vi "Load DAC Configuration.vi"(8 "error in":errorcluster, 10 "Config File refnum in":T1, 11 "DAC Keller Diff P 23X in":refnum<class "DAC Keller Diff P 23X.lvclass">) -> (0 "error out":errorcluster, 2 "Config File refnum out":T1, 3 "DAC Keller Diff P 23X out":refnum<class "DAC Keller Diff P 23X.lvclass">)   [LabVIEW 2019, in "DAC.lvlib" / "DAC Keller Diff P 23X.lvclass"]
uses:
  DAC Keller Diff P 23X.lvclass
  C:/Users/krio/Documents/LV_Projects/test-stand/App/DAC/DAC.lvclass
  <vilib>/Utility/config.llb/Config Data RefNum.ctl
  DAC.lvclass/DAC.ctl
  DAC Keller Diff P 23X.lvclass/DAC Keller Diff P 23X.ctl
  <vilib>/Utility/config.llb/Read Key (String).vi
  DAC.lvclass
  <vilib>/Utility/config.llb/NI_LVConfig.lvlib
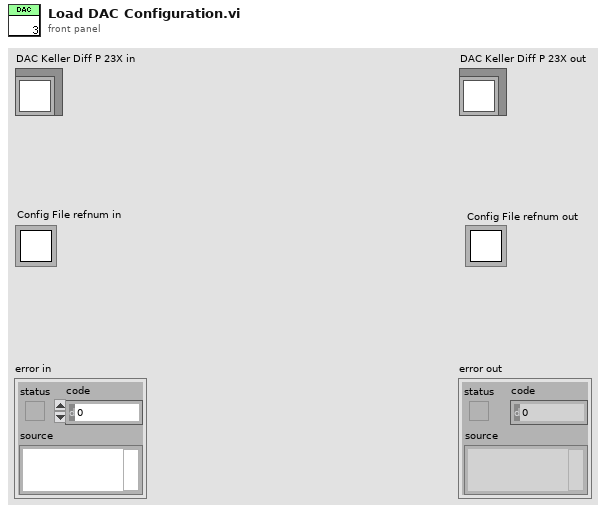
[diagram p1: front panel]
types:
  T1 = typedef "NI_LVConfig.lvlib/Config Data RefNum.ctl" = refnum<k1>
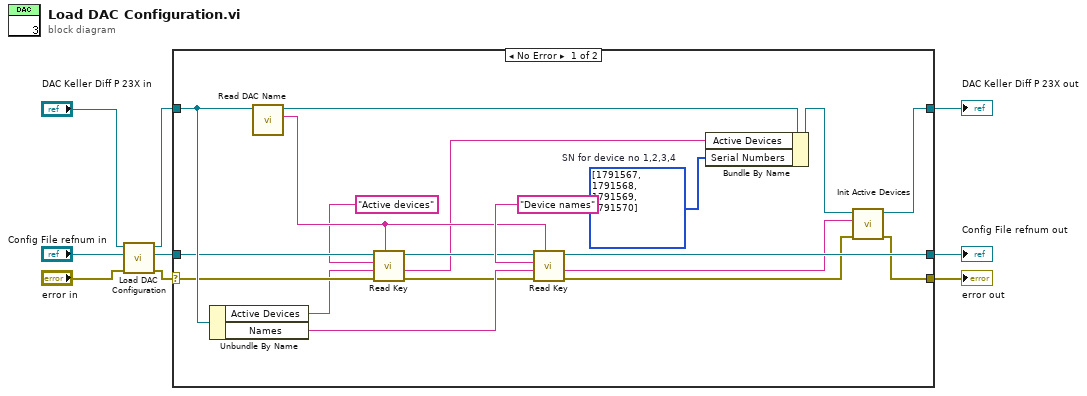
[diagram p0: block diagram]
diagram:
  n1 = call-parent "Load DAC Configuration.vi"("error in"="error in", "Config File refnum in"="Config File refnum in", "DAC in"="DAC Keller Diff P 23X in") -> ("error out"=w4:errorcluster, "Config File refnum out"=w5:T1, "DAC out"=w6:refnum<class "DAC Keller Diff P 23X.lvclass">)  [unwired: 6 in]
  n2 = case shown="No Error" w4 {
    selector: w4 -> [w18 w31]
    tunnel: [w20 w31] -> w1
    tunnel: [w23 w30] -> w3
    tunnel: w6 -> [w26 w30]
    tunnel: w5 -> [w16 w29]
    tunnel: [w28 w29] -> w2
    frame No Error {
      w10 = u32[] [1791567, 1791568, 1791569, 1791570]  # SN for device no 1,2,3,4
      n3 = Unbundle By Name(w26) -> ("Active Devices"=w13:string, "Names"=w25:string)
      n4 = call "Read DAC Name.vi"("DAC in"=w26) -> ("DAC Name"=w19:string, "DAC out"=w24:refnum<class "DAC Keller Diff P 23X.lvclass">)  [unwired: 8 in, 1 out]
      n5 = call-poly <vilib>:"Read Key.vi"("section"=w19, "error in (no error)"=w18, "default value"=w13, "key"="Active devices", "refnum"=w16) -> ("error out"=w17:errorcluster, "value"=w11:string, "refnum out"=w15:T1)  [unwired: 3 in, 1 out]
      n6 = call-poly <vilib>:"Read Key.vi"("section"=w19, "error in (no error)"=w17, "default value"=w25, "key"="Device names", "refnum"=w15) -> ("error out"=w21:errorcluster, "value"=w22:string, "refnum out"=w28:T1)  [unwired: 3 in, 1 out]
      n7 = Bundle By Name(cluster=w24, "Active Devices"=w11, "Serial Numbers"=w10) -> (w12:refnum<class "DAC Keller Diff P 23X.lvclass">)
      n8 = call "Init Active Devices.vi"("error in"=w21, "Device Names"=w22, "DAC Keller Diff P 23X in"=w12) -> ("error out"=w20:errorcluster, "DAC Keller Diff P 23X out"=w23:refnum<class "DAC Keller Diff P 23X.lvclass">)  [unwired: 7 in]
    }
    frame Error {
    }
  }
  "error out" <- w1
  "DAC Keller Diff P 23X out" <- w3
  "Config File refnum out" <- w2
